vi "TestMoveto.vi"(8 "error in (no error)":errorcluster) -> (0 "error out":errorcluster)   [LabVIEW 2019]
uses:
  PathCommands.Moveto/PathCommands.MoveTo.lvclass
  PathCommands/Point.ctl
  <vilib>/addons/_JKI Toolkits/Caraya/classes/Assert/Assert Equal Value_Variant.vi
  <vilib>/addons/_JKI Toolkits/Caraya/classes/Assert/Assert False.vi
  <vilib>/addons/_JKI Toolkits/Caraya/classes/Assert/Assert True.vi
  <vilib>/addons/_JKI Toolkits/Caraya/classes/Test/Test.lvclass
  PathCommands/PathCommands.lvclass
  <vilib>/addons/_JKI Toolkits/Caraya/classes/Assert/Assert.lvclass
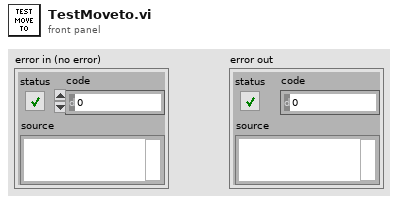
[diagram p1: front panel]
types:
  T1 = typedef "PathCommands.lvclass/Point.ctl" = cluster{"X":dbl, "Y":dbl}
  T2 = enum16{"None", "After", "Before", "Last", "First"}[]
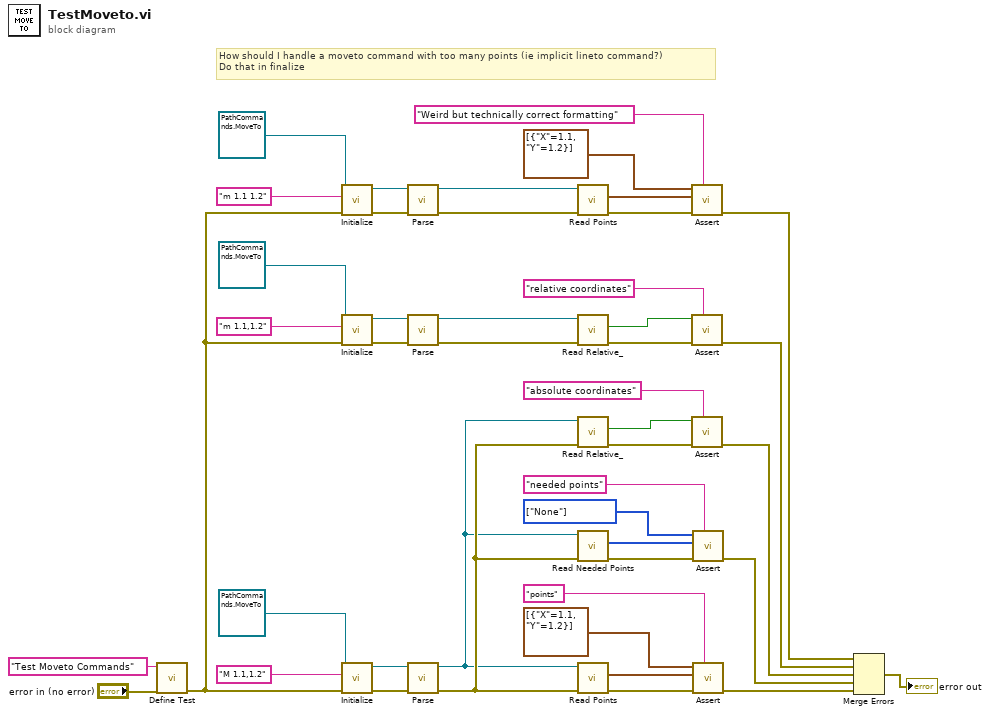
[diagram p0: block diagram]
diagram:
  w31 = T2 [enum."None"] items=["None", "After", "Before", "Last", "First"] ("Needed Points")
  # "How should I handle a moveto command with too many points (ie implicit lineto command?)\nDo that in finalize"
  n1 = call <vilib>:"Define Test.vi"("error in (no error)"="error in (no error)", "Label (VI Title)"="Test Moveto Commands") -> ("error out"=w7:errorcluster)  [unwired: 8 in, 1 out]
  n2 = call-dynamic "Initialize.vi"("error in (no error)"=w7, "CommandText"="m 1.1 1.2", "PathCommands.MoveTo in"=refnum<class "PathCommands.MoveTo.lvclass"> refnum ("PathCommands.MoveTo.lvclass")) -> ("error out"=w9:errorcluster, "PathCommands.MoveTo out"=w11:refnum<class "PathCommands.MoveTo.lvclass">)  [unwired: 7 in]
  n3 = call-dynamic "Initialize.vi"("error in (no error)"=w7, "CommandText"="m 1.1,1.2", "PathCommands.MoveTo in"=refnum<class "PathCommands.MoveTo.lvclass"> refnum ("PathCommands.MoveTo.lvclass")) -> ("error out"=w21:errorcluster, "PathCommands.MoveTo out"=w19:refnum<class "PathCommands.MoveTo.lvclass">)  [unwired: 7 in]
  n4 = call-dynamic "Initialize.vi"("error in (no error)"=w7, "CommandText"="M 1.1,1.2", "PathCommands.MoveTo in"=refnum<class "PathCommands.MoveTo.lvclass"> refnum ("PathCommands.MoveTo.lvclass")) -> ("error out"=w40:errorcluster, "PathCommands.MoveTo out"=w42:refnum<class "PathCommands.MoveTo.lvclass">)  [unwired: 7 in]
  n5 = call-dynamic "Parse.vi"("error in (no error)"=w9, "PathCommands.MoveTo in"=w11) -> ("error out"=w5:errorcluster, "PathCommands.MoveTo out"=w4:refnum<class "PathCommands.MoveTo.lvclass">)  [unwired: 8 in]
  n6 = call-dynamic "Parse.vi"("error in (no error)"=w21, "PathCommands.MoveTo in"=w19) -> ("error out"=w14:errorcluster, "PathCommands.MoveTo out"=w15:refnum<class "PathCommands.MoveTo.lvclass">)  [unwired: 8 in]
  n7 = call-dynamic "Parse.vi"("error in (no error)"=w40, "PathCommands.MoveTo in"=w42) -> ("error out"=w28:errorcluster, "PathCommands.MoveTo out"=w27:refnum<class "PathCommands.MoveTo.lvclass">)  [unwired: 8 in]
  n8 = call-dynamic "Read Points.vi"("error in (no error)"=w5, "PathCommands in"=w4) -> ("error out"=w3:errorcluster, "Points"=w2:T1[])  [unwired: 7 in, 1 out]
  n9 = call-dynamic "Read Relative_.vi"("error in (no error)"=w14, "PathCommands in"=w15) -> ("error out"=w16:errorcluster, "Relative?"=w17:bool)  [unwired: 7 in, 1 out]
  n10 = call-dynamic "Read Relative_.vi"("error in (no error)"=w28, "PathCommands in"=w27) -> ("error out"=w26:errorcluster, "Relative?"=w25:bool)  [unwired: 7 in, 1 out]
  n11 = call-dynamic "Read Needed Points.vi"("error in (no error)"=w28, "PathCommands in"=w27) -> ("error out"=w33:errorcluster, "Needed Points"=w32:T2)  [unwired: 7 in, 1 out]
  n12 = call-dynamic "Read Points.vi"("error in (no error)"=w28, "PathCommands in"=w27) -> ("error out"=w39:errorcluster, "Points"=w36:T1[])  [unwired: 7 in, 1 out]
  n13 = call-poly <vilib>:"Assert.vi"("Label"="Weird but technically correct formatting", "error in (no error)"=w3, "Y"=w2, "X"=T1[] [{"X"=1.1, "Y"=1.2}] ("Points")) -> ("error out"=w6:errorcluster)  [unwired: 6 in, 1 out]
  n14 = call-poly <vilib>:"Assert.vi"("Label"="relative coordinates", "error in (no error)"=w16, "True?"=w17) -> ("error out"=w13:errorcluster)  [unwired: 7 in, 1 out]
  n15 = call-poly <vilib>:"Assert.vi"("Label"="absolute coordinates", "error in (no error)"=w26, "False?"=w25) -> ("error out"=w23:errorcluster)  [unwired: 7 in, 1 out]
  n16 = call-poly <vilib>:"Assert.vi"("Label"="needed points", "error in (no error)"=w33, "Y"=w32, "X"=w31) -> ("error out"=w29:errorcluster)  [unwired: 6 in, 1 out]
  n17 = call-poly <vilib>:"Assert.vi"("Label"="points", "error in (no error)"=w39, "Y"=w36, "X"=T1[] [{"X"=1.1, "Y"=1.2}] ("Points")) -> ("error out"=w37:errorcluster)  [unwired: 6 in, 1 out]
  n18 = Merge Errors(w6, w13, w23, w29, w37) -> (→"error out":errorcluster)
